vi "IMU_serial_Write_Read.vi"(6 "Delay (ms)":u32, 7 "Command Selection":u16(ring) items=["MSP_IDENT", "MSP_STATUS", "MSP_RAW_IMU", "MSP_RAW_GPS", "MSP_ATTITUDE", "MSP_ALTITUDE", "MSP_ACC_CALIBRATION", "MSP_MAG_CALIBRATION"], 8 "error in (no error)":errorcluster caption="Fehler (Eingang, kein Fehler)", 11 "VISA resource name IN":refnum<visa-resource-name>) -> (0 "error IO":errorcluster, 2 "Received Raw Data Byte-Array U8":u8[](array[numeric]), 3 "VISA resource name OUT":refnum<visa-resource-name>)   [LabVIEW 2017]
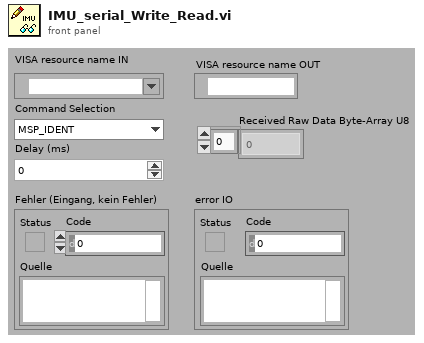
[diagram p1: front panel]
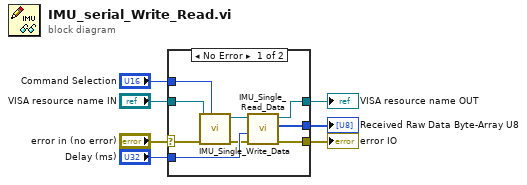
[diagram p0: block diagram]
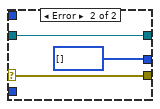
[diagram p2: hidden frame]
diagram:
  n1 = case shown="No Error" "error in (no error)" {
    selector: "error in (no error)" -> [w9 w19]
    tunnel: "VISA resource name IN" -> [w16 w18]
    tunnel: "Command Selection" -> [w15 _]
    tunnel: "Delay (ms)" -> [w14 _]
    tunnel: [w13 w18] -> w4
    tunnel: [w12 u8[] [] ("Received Raw Data Byte-Array U8 2")] -> w3
    tunnel: [w8 w19] -> w2
    frame No Error {
      n2 = call "IMU_Single_Write_Data.vi"("Command Selection"=w15, "error in (no error)"=w9, "VISA resource name IN"=w16) -> ("error out"=w10:errorcluster, "VISA resource name OUT"=w11:refnum<visa-resource-name>)  [unwired: 7 in]
      n3 = call "IMU_Single_Read_Data.vi"("error in (no error)"=w10, "Delay (ms)"=w14, "VISA resource name IN"=w11) -> ("error out"=w8:errorcluster, "Received Raw Data Byte-Array U8"=w12:u8[], "VISA resource name OUT"=w13:refnum<visa-resource-name>)  [unwired: 6 in]
    }
    frame Error {
    }
  }
  "Received Raw Data Byte-Array U8" <- w3
  "VISA resource name OUT" <- w4
  "error IO" <- w2
